vi "ZCAN_SetSendMode.vi"(8 "error in (no error)":errorcluster, 9 "SendMode":enum16{"Normal Mode", "Dueue Mode"}(ring), 10 "CH_ID":i32, 11 "DeviceHANDLE":u32) -> (0 "error out":errorcluster)   [LabVIEW 2020, in "zlgcan.lvlib"]
doc: "设置发送模式，0，正常发送 ，1 队列发送"
uses:
  zlgcan.lvlib
  bin/zlgcan_wrap.dll
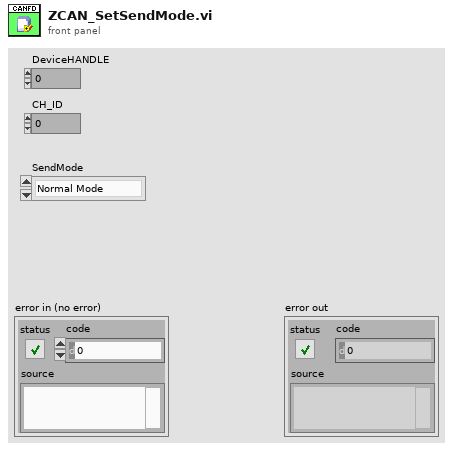
[diagram p1: front panel]
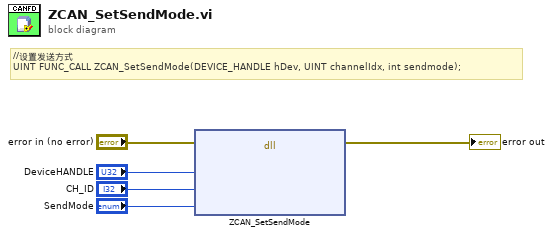
[diagram p0: block diagram]
diagram:
  # "//设置发送方式\nUINT FUNC_CALL ZCAN_SetSendMode(DEVICE_HANDLE hDev, UINT channelIdx, int sendmode);"
  n1 = dll-call lib="E:/Jabil tools/JabilTestLib/LV/ZLG_CANFD/bin/zlgcan_wrap.dll" fn="ZCAN_SetSendMode"(error in="error in (no error)", "DeviceHANDLE"="DeviceHANDLE", "CH_ID"="CH_ID", "SendMode"="SendMode") -> (error out=→"error out":errorcluster)  [unwired: 6 in, 1 out]
